vi "GenericJoystickCalibrate.vi"(4 "Raw Joystick Value":dbl, 5 "Maximum":dbl(slide)=1.0 min=0.6 max=1.0 scale=0.6..1.0, 6 "Minimum":dbl(slide)=-1.0 min=-1.0 max=-0.6 scale=-1.0..-0.6, 7 "Deadband":dbl(slide) min=0.0 max=0.4 scale=0.0..0.4) -> (0 "Scaled Joystick Value":dbl format="%.2g")   [LabVIEW 2020]
doc: "This VI applies calibration values (deadband, min, and max) to a generic joystick axis and rescales the output to range from [-1,+1]."
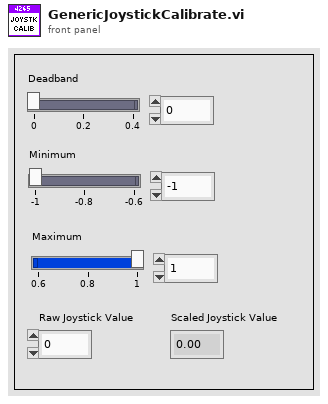
[diagram p1: front panel]
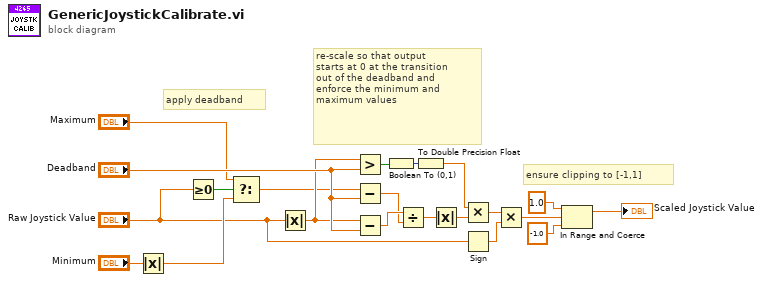
[diagram p0: block diagram]
diagram:
  # "ensure clipping to [-1,1]"
  # "re-scale so that output\nstarts at 0 at the transition\nout of the deadband and\nenforce the minimum and\nmaximum values"
  # "apply deadband"
  n1 = Absolute Value(x="Minimum") -> (abs(x)=w5:dbl)
  n2 = Greater Or Equal To 0?(x="Raw Joystick Value") -> (x >= 0?=w9:bool)
  n3 = Select(t="Maximum", s=w9, f=w5) -> (s? t:f=w6:dbl)
  n4 = Absolute Value(x="Raw Joystick Value") -> (abs(x)=w13:dbl)
  n5 = Greater?(x=w13, y="Deadband") -> (0:w12:bool)
  n6 = Subtract(x=w6, y="Deadband") -> (x-y=w16:dbl)
  n7 = Subtract(x=w13, y="Deadband") -> (x-y=w17:dbl)
  n8 = Boolean To (0,1)(Boolean=w12) -> (0, 1=w19:i16)
  n9 = Divide(x=w17, y=w16) -> (x/y=w15:dbl)
  n10 = To Double Precision Float(number=w19) -> (double precision float=w18:dbl)
  n11 = Absolute Value(x=w15) -> (abs(x)=w3:dbl)
  n12 = Multiply(x=w18, y=w3) -> (x*y=w20:dbl)
  n13 = Sign(1:"Raw Joystick Value") -> (0:w14:dbl)
  n14 = Multiply(x=w20, y=w14) -> (x*y=w4:dbl)
  n15 = In Range and Coerce(upper limit=1.0, x=w4, lower limit=-1.0) -> (coerced(x)=→"Scaled Joystick Value":dbl)  [unwired: 1 out]
